vi "Get Telemetry.vi"(8 "error in (no error)":errorcluster, 11 "S4GUI in":refnum<class "S4GUI.lvclass">) -> (0 "error out":errorcluster, 3 "S4GUI out":refnum<class "S4GUI.lvclass">)   [LabVIEW 2018, in "S4GUI.lvclass"]
uses:
  S4GUI.lvclass
  S4GUI.lvclass/S4GUI.ctl
  Instrument/Instrument.lvclass/Instrument.ctl
  Device/Optics/Optics.lvclass/Optics.ctl
  Device/Optics/Opt_Selector/Opt_Selector.lvclass
  Device/Optics/Opt_Continuous/Opt_Continuous.lvclass
  TCS/TCS.lvclass
  TelFocus/TelFocus.lvclass
  WeatherStation/WeatherStation.lvclass
  WeatherSensor/WeatherSensor.lvclass
  SecMirror/SecMirror.lvclass
  Telemetry/Telemetry.lvclass
  Instrument/Instrument.lvclass
  Device/Optics/Optics.lvclass
panel:
  out "ICS header":string
  out "unsigned byte array":u8[](array[numeric])
  in  "TCS str":string
  out "SD":string
  out "JD":string
  out "OBJ":string
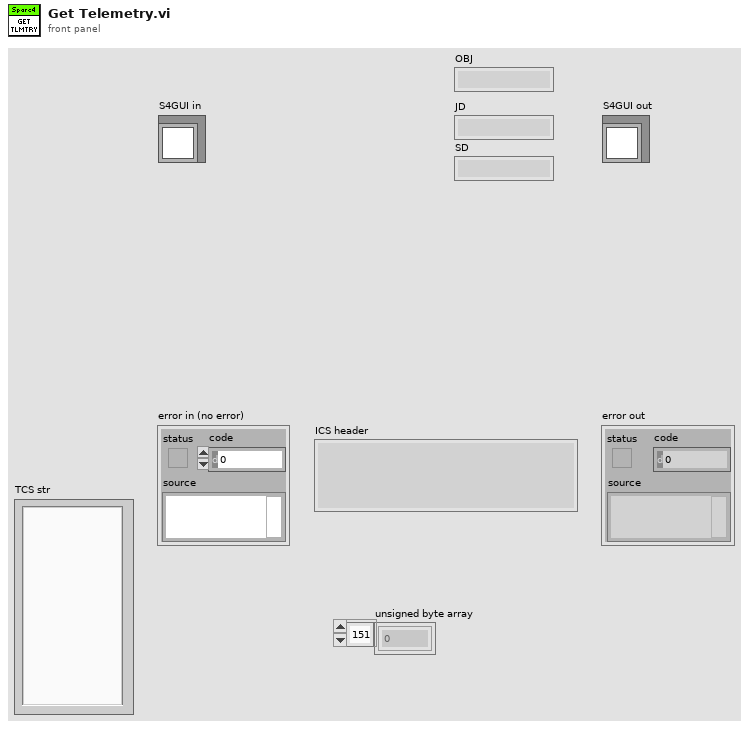
[diagram p1: front panel]
types:
  T1 = cluster{"broker":string, "version":string, "date":string, "hour":string, "outHumidity":string, "intHumidity":string, "inTemp":string, "outTemp":string, "windSpeed":string, "windDirection":string, "pressure":string, "dewOut":string, "dewIn":string, "leaf":string, "rain":string, "windChill":string}
  T2 = cluster{"broker":string, "version":string, "objectName":string, "raAcquis":string, "decAcquis":string, "epochAcquis":string, "airMass":string, "julianDate":string, "sideralTime":string, "hourAngle":string, "date":string, "time":string, "rightAscention":string, "declination":string, "guideStr":string, "guideAng":string, "guideNor":string, "guideEsp":string, "guideCas":string, "guidePlaca":string, "statShutter":string, "posCup":string, "raOnTarget":bool, "decOnTarget":bool, "dome":bool, "domeOnTarget":bool, "guider":bool, "mount":bool, "grossMovement":bool, "fimeMovement":bool, "objCentrado":bool, "varTracking":bool, "shutter":bool, "cmd":string}
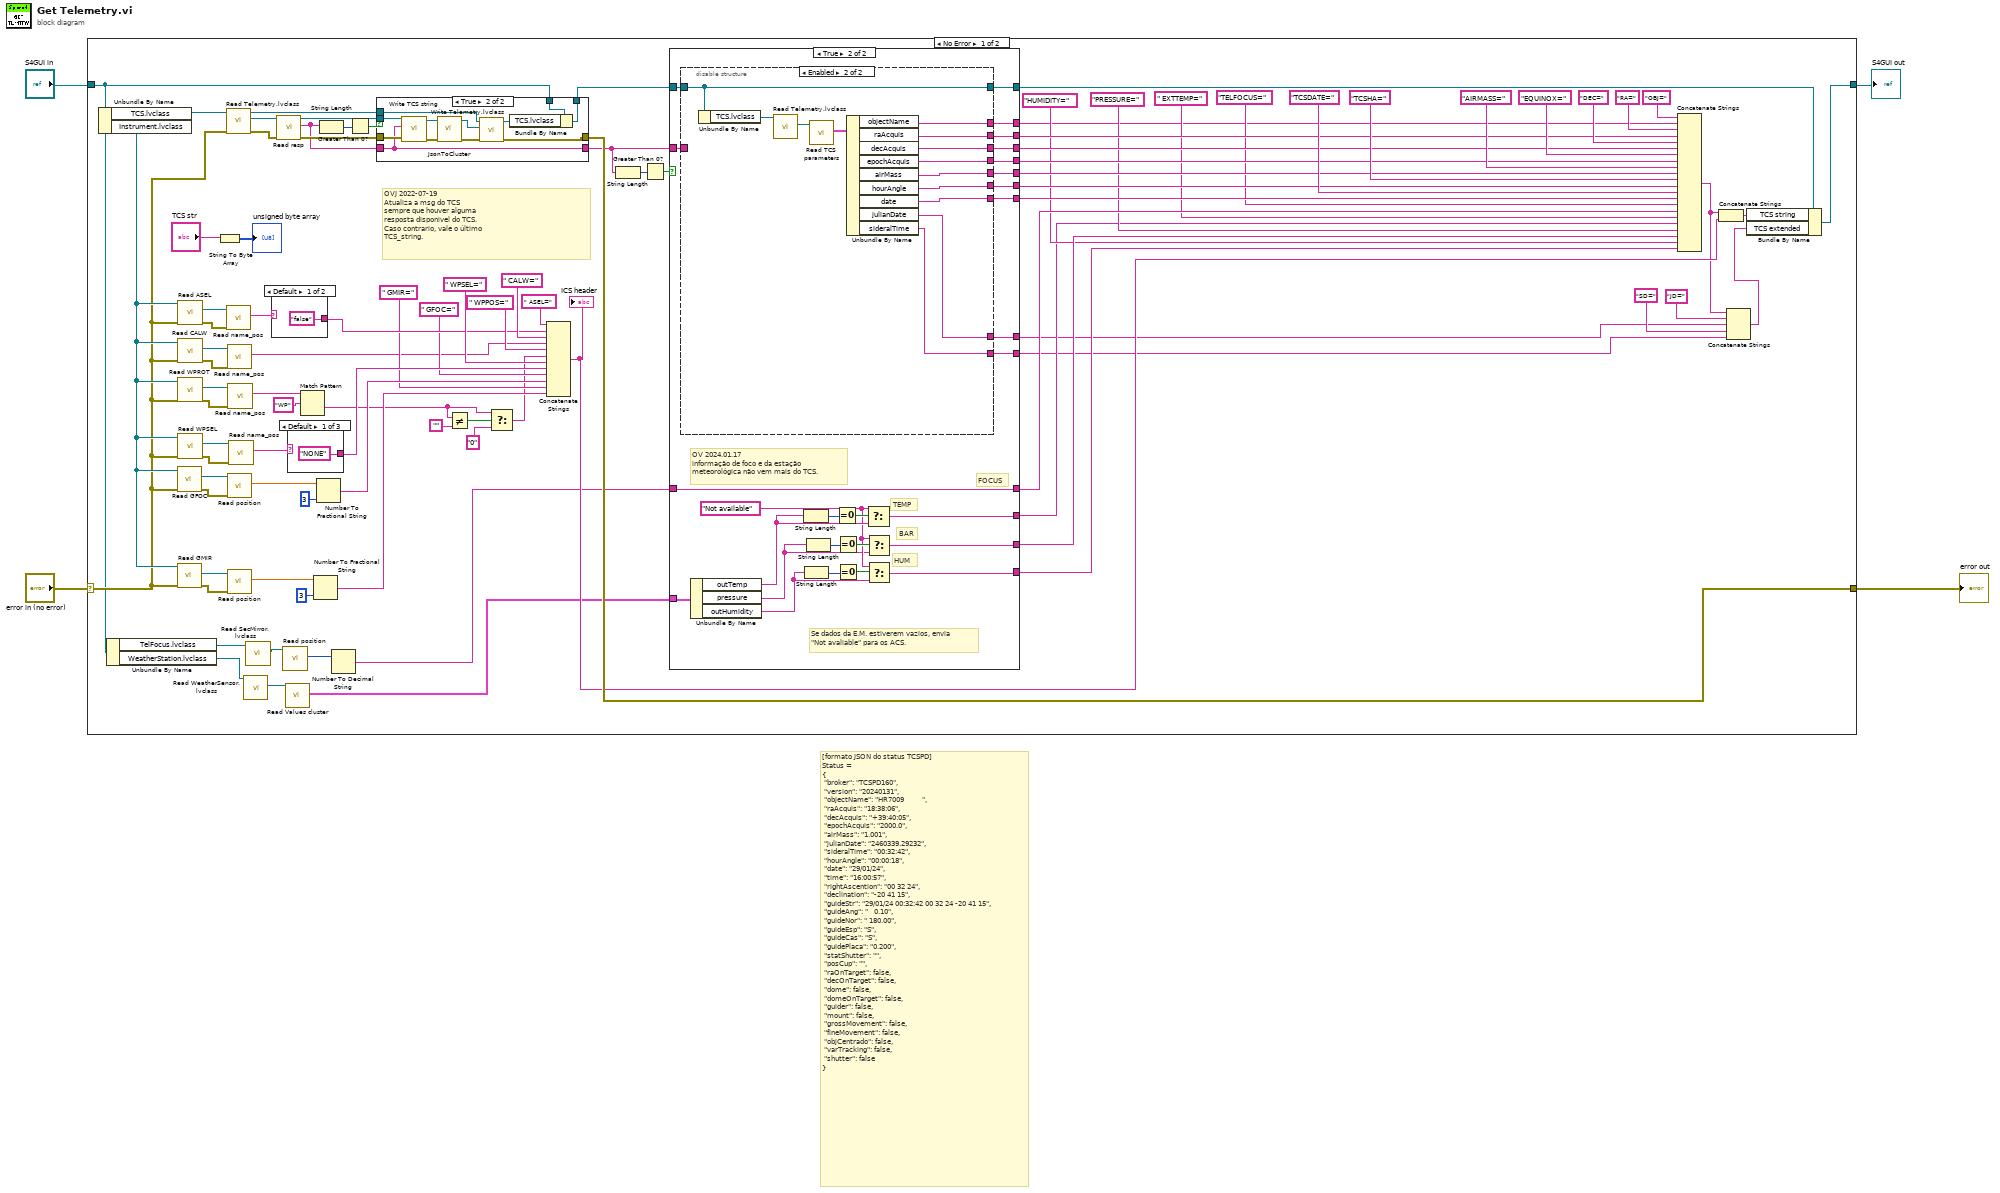
[diagram p0: block diagram]
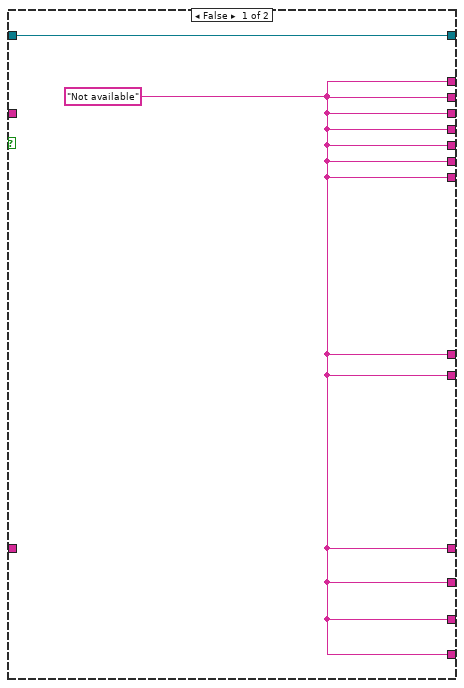
[diagram p2: hidden frame]
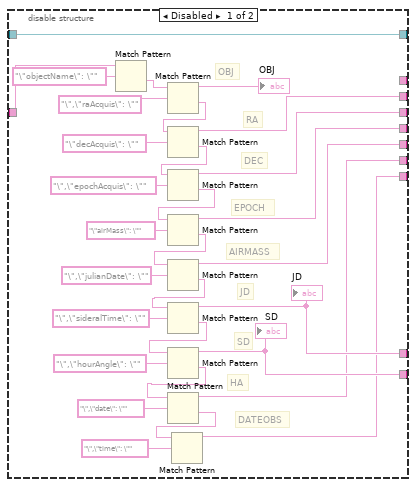
[diagram p3: hidden frame]
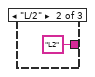
[diagram p4: hidden frame]
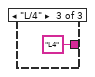
[diagram p5: hidden frame]
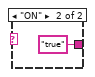
[diagram p6: hidden frame]
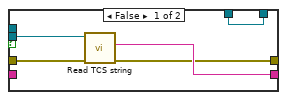
[diagram p7: hidden frame]
diagram:
  # "[formato JSON do status TCSPD]\nStatus =\n{\n\t\"broker\": \"TCSPD160\",\n\t\"version\": \"20240131\",\n\t\"objectName\": \"HR7009         \",\n\t\"raAcquis\": \"18:38:06\",\n\t\"decAcquis\": \"+39:40:05\",\n\t\"epochAcquis\": \"2000.0\",\n\t\"airMass\": \"1.001\",\n\t\"julianDate\": \"2460339.29232\",\n\t\"sideralTime\": \"00:32:42\",\n\t\"hourAngle\": \"00:00:18\",\n\t\"date\": \"29/01/24\",\n\t\"time\": \"16:00:57\",\n\t\"rightAscention\": \"00 32 24\",\n\t\"declination\": \"-20 41 15\",\n\t\"guideStr\": \"29/01/24 00:32:42 00 32 24 -20 41 15\",\n\t\"guideAng\": \"   0.10\",\n\t\"guideNor\": \" 180.00\",\n\t\"guideEsp\": \"S\",\n\t\"guideCas\": \"S\",\n\t\"guidePlaca\": \"0.200\",\n\t\"statShutter\": \"\",\n\t\"posCup\": \"\",\n\t\"raOnTarget\": false,\n\t\"decOnTarget\": false,\n\t\"dome\": false,\n\t\"domeOnTarget\": false,\n\t\"guider\": false,\n\t\"mount\": false,\n\t\"grossMovement\": false,\n\t\"fineMovement\": false,\n\t\"objCentrado\": false,\n\t\"varTracking\": false,\n\t\"shutter\": false\n}"
  n1 = case shown="No Error" "error in (no error)" {
    selector: "error in (no error)" -> [w66 w194]
    tunnel: [w85 w194] -> w3
    tunnel: [w26 w193] -> w1
    tunnel: "S4GUI in" -> [w16 w193]
    frame No Error {
      # "OVJ 2022-07-19\nAtualiza a msg do TCS\nsempre que houver alguma\nresposta disponivel do TCS.\nCaso contrario, vale o último\nTCS_string."
      n2 = Unbundle By Name(w16) -> ("TCS.lvclass"=w98:refnum<class "TCS.lvclass">, "Instrument.lvclass"=w67:refnum<class "Instrument.lvclass">)
      n3 = Unbundle By Name(w16) -> ("TelFocus.lvclass"=w15:refnum<class "TelFocus.lvclass">, "WeatherStation.lvclass"=w11:refnum<class "WeatherStation.lvclass">)
      n4 = call "Read GFOC.vi"("error in (no error)"=w66, "Instrument in"=w67) -> ("error out"=w55:errorcluster, "Opt_Continuous.lvclass"=w61:refnum<class "Opt_Continuous.lvclass">)  [unwired: 7 in, 1 out]
      n5 = call "Read GMIR.vi"("error in (no error)"=w66, "Instrument in"=w67) -> ("error out"=w54:errorcluster, "Opt_Continuous.lvclass"=w60:refnum<class "Opt_Continuous.lvclass">)  [unwired: 7 in, 1 out]
      n6 = call "Read ASEL.vi"("error in (no error)"=w66, "Instrument in"=w67) -> ("error out"=w59:errorcluster, "Opt_Selector.lvclass"=w65:refnum<class "Opt_Selector.lvclass">)  [unwired: 7 in, 1 out]
      n7 = call "Read CALW.vi"("error in (no error)"=w66, "Instrument in"=w67) -> ("error out"=w58:errorcluster, "Opt_Selector.lvclass"=w64:refnum<class "Opt_Selector.lvclass">)  [unwired: 7 in, 1 out]
      n8 = call "Read WPROT.vi"("error in (no error)"=w66, "Instrument in"=w67) -> ("error out"=w57:errorcluster, "Opt_Selector.lvclass"=w63:refnum<class "Opt_Selector.lvclass">)  [unwired: 7 in, 1 out]
      n9 = call "Read WPSEL.vi"("error in (no error)"=w66, "Instrument in"=w67) -> ("error out"=w56:errorcluster, "Opt_Selector.lvclass"=w62:refnum<class "Opt_Selector.lvclass">)  [unwired: 7 in, 1 out]
      n10 = String To Byte Array(string="TCS str") -> (unsigned byte array=→"unsigned byte array":u8[])
      n11 = call-dynamic "Read Telemetry.lvclass.vi"("error in (no error)"=w66, "TCS in"=w98) -> ("error out"=w83:errorcluster, "Telemetry.lvclass"=w84:refnum<class "Telemetry.lvclass">, "TCS out"=w77:refnum<class "TCS.lvclass">)  [unwired: 7 in]
      n12 = call "Read name_pos.vi"("error in (no error)"=w59, "Optics in"=w65) -> ("name_pos"=w47:string)  [unwired: 7 in, 2 out]
      n13 = call "Read name_pos.vi"("error in (no error)"=w58, "Optics in"=w64) -> ("name_pos"=w17:string)  [unwired: 7 in, 2 out]
      n14 = call "Read position.vi"("error in (no error)"=w55, "Optics in"=w61) -> ("position"=w41:dbl)  [unwired: 7 in, 2 out]
      n15 = call "Read position.vi"("error in (no error)"=w54, "Optics in"=w60) -> ("position"=w37:dbl)  [unwired: 7 in, 2 out]
      n16 = call "Read name_pos.vi"("error in (no error)"=w57, "Optics in"=w63) -> ("name_pos"=w49:string)  [unwired: 7 in, 2 out]
      n17 = call "Read name_pos.vi"("error in (no error)"=w56, "Optics in"=w62) -> ("name_pos"=w45:string)  [unwired: 7 in, 2 out]
      n18 = call-dynamic "Read WeatherSensor.lvclass.vi"("WeatherStation in"=w11) -> ("WeatherSensor.lvclass"=w10:refnum<class "WeatherSensor.lvclass">)  [unwired: 8 in, 2 out]
      n19 = call-dynamic "Read SecMirror.lvclass.vi"("TelFocus in"=w15) -> ("SecMirror.lvclass"=w14:refnum<class "SecMirror.lvclass">)  [unwired: 8 in, 2 out]
      n20 = case shown="Default" w47 {
        tunnel: ["false" ("regular expression") "true" ("regular expression")] -> w46
        frame Default {
        }
        frame "ON" {
        }
      }
      n21 = call-dynamic "Read resp.vi"("error in (no error)"=w83, "Device in"=w84) -> ("error out"=w82:errorcluster, "resp"=w78:string, "Device out"=w79:refnum<class "Telemetry.lvclass">)  [unwired: 7 in]
      n22 = call-dynamic "Read position.vi"("SecMirror in"=w14) -> ("position"=w13:i32)  [unwired: 8 in, 2 out]
      n23 = call-dynamic "Read Values cluster.vi"("WeatherSensor in"=w10) -> ("Values cluster"=w9:T1)  [unwired: 8 in, 2 out]
      n24 = case shown="Default" w45 {
        tunnel: ["NONE" ("regular expression") "L2" ("regular expression") "L4" ("regular expression")] -> w44
        frame Default {
        }
        frame "L/2" {
        }
        frame "L/4" {
        }
      }
      n25 = Match Pattern(string=w49, regular expression="WP") -> (after substring=w30:string)  [unwired: 1 in, 3 out]
      n26 = Number To Fractional String(number=w37, precision (6)=i16 3) -> (F-format string=w36:string)  [unwired: 2 in]
      n27 = Number To Fractional String(number=w41, precision (6)=i16 3) -> (F-format string=w40:string)  [unwired: 2 in]
      n28 = String Length(string=w78) -> (length=w81:i32)
      n29 = Number To Decimal String(number=w13) -> (decimal integer string=w12:string)  [unwired: 1 in]
      n30 = Greater Than 0?(x=w81) -> (x > 0?=w80:bool)
      n31 = case shown="True" w80 {
        tunnel: [w180 w190] -> w33
        tunnel: [w179 w182] -> w85
        tunnel: w82 -> [w178 w192]
        tunnel: w79 -> [w177 w191]
        tunnel: w78 -> [_ w190]
        tunnel: w16 -> [w176 w189]
        tunnel: w77 -> [_ w188]
        tunnel: [w176 w186] -> w8
        frame False {
          n32 = call-dynamic "Read TCS string.vi"("error in (no error)"=w178, "Telemetry in"=w177) -> ("error out"=w179:errorcluster, "TCS string"=w180:string)  [unwired: 7 in, 1 out]
        }
        frame True {
          n33 = call-dynamic "Write TCS string.vi"("error in (no error)"=w192, "TCS string"=w190, "Telemetry in"=w191) -> ("error out"=w184:errorcluster, "Telemetry out"=w185:refnum<class "Telemetry.lvclass">)  [unwired: 7 in]
          n34 = call-dynamic "JsonToCluster.vi"("error in (no error)"=w184, "Telemetry in"=w185) -> ("error out"=w181:errorcluster, "Telemetry out"=w183:refnum<class "Telemetry.lvclass">)  [unwired: 8 in]
          n35 = call-dynamic "Write Telemetry.lvclass.vi"("error in (no error)"=w181, "Telemetry.lvclass"=w183, "TCS in"=w188) -> ("error out"=w182:errorcluster, "TCS out"=w187:refnum<class "TCS.lvclass">)  [unwired: 7 in]
          n36 = Bundle By Name(cluster=w189, "TCS.lvclass"=w187) -> (w186:refnum<class "S4GUI.lvclass">)
        }
      }
      n37 = Not Equal?(x=w30, y="") -> (x != y?=w31:bool)
      n38 = Select(t=w30, s=w31, f="0") -> (s? t:f=w28:string)
      n39 = Concatenate Strings(" ASEL=" ("string"), w46, " CALW=" ("string"), w17, " WPPOS=" ("string"), w28, " WPSEL=" ("string"), w44, " GFOC=" ("string"), w40, " GMIR=" ("string"), w36) -> (w25:string)
      "ICS header" <- w25
      n40 = String Length(string=w33) -> (length=w34:i32)
      n41 = Greater Than 0?(x=w34) -> (x > 0?=w35:bool)
      n42 = case shown="True" w35 {
        tunnel: [w99 w111] -> w91
        tunnel: [w99 w110] -> w90
        tunnel: [w99 w109] -> w89
        tunnel: [w99 w108] -> w88
        tunnel: [w99 w105] -> w87
        tunnel: [w99 w104] -> w86
        tunnel: [w99 w127] -> w75
        tunnel: [w99 w116] -> w70
        tunnel: [w99 w113] -> w68
        tunnel: w33 -> [_ w112]
        tunnel: [w99 w123] -> w27
        tunnel: [w99 w107] -> w20
        tunnel: [w99 w106] -> w19
        tunnel: w12 -> [_ w127]
        tunnel: w9 -> [_ w126]
        tunnel: w8 -> [w100 w103]
        tunnel: [w100 w102] -> w7
        tunnel: [w99 w101] -> w5
        frame False {
          w99 = "Not available" ("t")
        }
        frame True {
          w117 = "Not available" ("t")
          # "Se dados da E.M. estiverem vazios, envia\n\"Not avaliable\" para os ACS."
          # "OV 2024.01.17\ninformação de foco e da estação\nmeteorológica não vem mais do TCS."
          # "HUM"
          # "BAR"
          # "TEMP"
          # "FOCUS"
          n43 = disable-structure shown="Enabled" {
            disable-tunnel: w112 -> [w157 _]
            disable-tunnel: [w150 w166] -> w111
            disable-tunnel: [w147 w165] -> w110
            disable-tunnel: [w144 w164] -> w109
            disable-tunnel: [w142 w163] -> w108
            disable-tunnel: [w139 w160] -> w107
            disable-tunnel: [w136 w159] -> w106
            disable-tunnel: [w132 w162] -> w105
            disable-tunnel: [w129 w161] -> w104
            disable-tunnel: w103 -> [w128 w167]
            disable-tunnel: [w128 w167] -> w102
            disable-tunnel: [_ w158] -> w101
            frame Disabled {
              # "DATEOBS"
              # "HA"
              # "SD"
              # "JD"
              # "AIRMASS"
              # "EPOCH"
              # "DEC"
              # "RA"
              # "OBJ"
              n44 = Match Pattern(string=w157, regular expression="\"objectName\": \"") -> (after substring=w156:string)  [unwired: 1 in, 3 out]
              n45 = Match Pattern(string=w156, regular expression="\",\"raAcquis\": \"") -> (before substring=→"OBJ":string, after substring=w152:string)  [unwired: 1 in, 2 out]
              n46 = Match Pattern(string=w152, regular expression="\"decAcquis\": \"") -> (before substring=w150:string, after substring=w148:string)  [unwired: 1 in, 2 out]
              n47 = Match Pattern(string=w148, regular expression="\",\"epochAcquis\": \"") -> (before substring=w147:string, after substring=w145:string)  [unwired: 1 in, 2 out]
              n48 = Match Pattern(string=w145, regular expression="\"airMass\": \"") -> (before substring=w144:string, after substring=w135:string)  [unwired: 1 in, 2 out]
              n49 = Match Pattern(string=w135, regular expression="\",\"julianDate\": \"") -> (before substring=w142:string, after substring=w140:string)  [unwired: 1 in, 2 out]
              n50 = Match Pattern(string=w140, regular expression="\",\"sideralTime\": \"") -> (before substring=w139:string, after substring=w137:string)  [unwired: 1 in, 2 out]
              "JD" <- w139
              n51 = Match Pattern(string=w137, regular expression="\",\"hourAngle\": \"") -> (before substring=w136:string, after substring=w133:string)  [unwired: 1 in, 2 out]
              "SD" <- w136
              n52 = Match Pattern(string=w133, regular expression="\",\"date\": \"") -> (before substring=w132:string, after substring=w130:string)  [unwired: 1 in, 2 out]
              n53 = Match Pattern(string=w130, regular expression="\",\"time\": \"") -> (before substring=w129:string)  [unwired: 1 in, 3 out]
            }
            frame Enabled {
              n54 = Unbundle By Name(w167) -> ("TCS.lvclass"=w170:refnum<class "TCS.lvclass">)
              n55 = call-dynamic "Read Telemetry.lvclass.vi"("TCS in"=w170) -> ("Telemetry.lvclass"=w169:refnum<class "Telemetry.lvclass">)  [unwired: 8 in, 2 out]
              n56 = call-dynamic "Read TCS parameters.vi"("Telemetry in"=w169) -> ("TCS parameters"=w168:T2)  [unwired: 8 in, 2 out]
              n57 = Unbundle By Name(w168) -> ("objectName"=w158:string, "raAcquis"=w166:string, "decAcquis"=w165:string, "epochAcquis"=w164:string, "airMass"=w163:string, "hourAngle"=w162:string, "date"=w161:string, "julianDate"=w160:string, "sideralTime"=w159:string)
            }
          }
          n58 = Unbundle By Name(w126) -> ("outTemp"=w122:string, "pressure"=w115:string, "outHumidity"=w114:string)
          n59 = String Length(string=w122) -> (length=w125:i32)
          n60 = String Length(string=w114) -> (length=w119:i32)
          n61 = String Length(string=w115) -> (length=w121:i32)
          n62 = Equal To 0?(x=w125) -> (x = 0?=w124:bool)
          n63 = Equal To 0?(x=w121) -> (x = 0?=w120:bool)
          n64 = Equal To 0?(x=w119) -> (x = 0?=w118:bool)
          n65 = Select(t=w117, s=w124, f=w122) -> (s? t:f=w123:string)
          n66 = Select(t=w117, s=w120, f=w115) -> (s? t:f=w116:string)
          n67 = Select(t=w117, s=w118, f=w114) -> (s? t:f=w113:string)
        }
      }
      n68 = Concatenate Strings("OBJ=" ("string"), w5, "RA=" ("string"), w91, "DEC=" ("string"), w90, "EQUINOX=" ("string"), w89, "AIRMASS=" ("string"), w88, "TCSHA=" ("string"), w87, "TCSDATE=" ("string"), w86, "TELFOCUS=" ("string"), w75, " EXTTEMP=" ("string"), w27, "PRESSURE=" ("string"), w70, "HUMIDITY=" ("string"), w68) -> (w23:string)
      n69 = Concatenate Strings(w23, w25) -> (w24:string)
      n70 = Concatenate Strings(w23, "JD=" ("string"), w20, "SD=" ("string"), w19) -> (w18:string)
      n71 = Bundle By Name(cluster=w7, "TCS string"=w24, "TCS extended"=w18) -> (w26:refnum<class "S4GUI.lvclass">)
    }
    frame Error {
    }
  }
  "error out" <- w3
  "S4GUI out" <- w1
